vi "SBG_Ellipse_init_UART (SubVI).vi"(10 "Baudrate":u32, 11 "VISA Refnum in":refnum<visa-resource-name>) -> (0 "error out":errorcluster, 3 "VISA Refnum out":refnum<visa-resource-name>)   [LabVIEW 2018]
uses:
  <vilib>/Instr/_visa.llb/VISA Configure Serial Port (Instr).vi
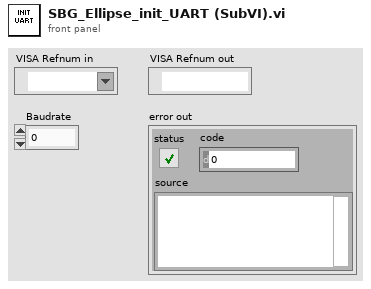
[diagram p1: front panel]
types:
  T1 = cluster{"baud rate (9600)":u32, "data bits (8)":u16, "parity (0:none)":enum16{"None", "Odd", "Even", "Mark", "Space"}, "stop bits (10: 1 bit)":u16, "flow control (0:none)":u16, "termination char\n(0xA = '\\n' = LF) ":u8, "Enable Termination\nChar (T)":bool, "timeout (10sec)":u32}
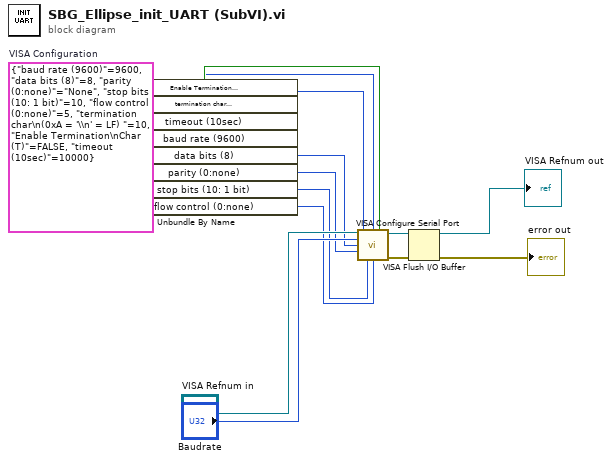
[diagram p0: block diagram]
diagram:
  w7 = T1 {"baud rate (9600)"=9600, "data bits (8)"=8, "parity (0:none)"=enum."None", "stop bits (10: 1 bit)"=10, "flow control (0:none)"=5, "termination char\n(0xA = '\\n' = LF) "=10, "Enable Termination\nChar (T)"=FALSE, "timeout (10sec)"=10000}  # VISA Configuration
  n1 = Unbundle By Name(w7) -> ("Enable Termination\nChar (T)"=w6:bool, "termination char\n(0xA = '\\n' = LF)"=w5:u8, "timeout (10sec)"=w4:u32, "data bits (8)"=w8:u16, "parity (0:none)"=w1:enum16{"None", "Odd", "Even", "Mark", "Space"}, "stop bits (10: 1 bit)"=w2:u16, "flow control (0:none)"=w3:u16)  [unwired: 1 out]
  n2 = call-poly "VISA Configure Serial Port"("VISA resource name"="VISA Refnum in", "timeout (10sec)"=w4, "termination char\n(0xA = '\\n' = LF)"=w5, "Enable Termination\nChar (T)"=w6, "baud rate (9600)"="Baudrate", "data bits (8)"=w8, "parity (0:none)"=w1, "stop bits (10: 1 bit)"=w2, "flow control (0:none)"=w3) -> ("VISA resource name out"=w11:refnum<visa-resource-name>, "error out"=w12:errorcluster)  [unwired: 5 in]
  n3 = VISA Flush I/O Buffer(VISA resource name=w11, error in (no error)=w12) -> (VISA resource name out=→"VISA Refnum out":refnum<visa-resource-name>, error out=→"error out":errorcluster)  [unwired: 1 in]
